vi "Main.vi"() -> ()   [LabVIEW 2020]
uses:
  <vilib>/userdefined/High Color/IMAQdx.ctl
panel:
  out "# of Matches":i32
  out "Error Out":errorcluster
  in  "Start":bool
  in  "Stop":bool
  out "# Iter":i32
  out "Image":T1(plugin-control)
  in  "Inspection Part":enum32{"P2", "P3 Top", "P3 Side"}(tab)
  out "P2 Hole":sgl
  out "P2 Left Edge Angle":sgl
  out "P2 Right Edge Angle":sgl
  out "P2 Hole Status":bool
  out "P2 Left Edge Angle Status":bool
  out "P2 Right Edge Angle Status":bool
  out "P2 Status":bool
  # "Smart Vision System Testbench"
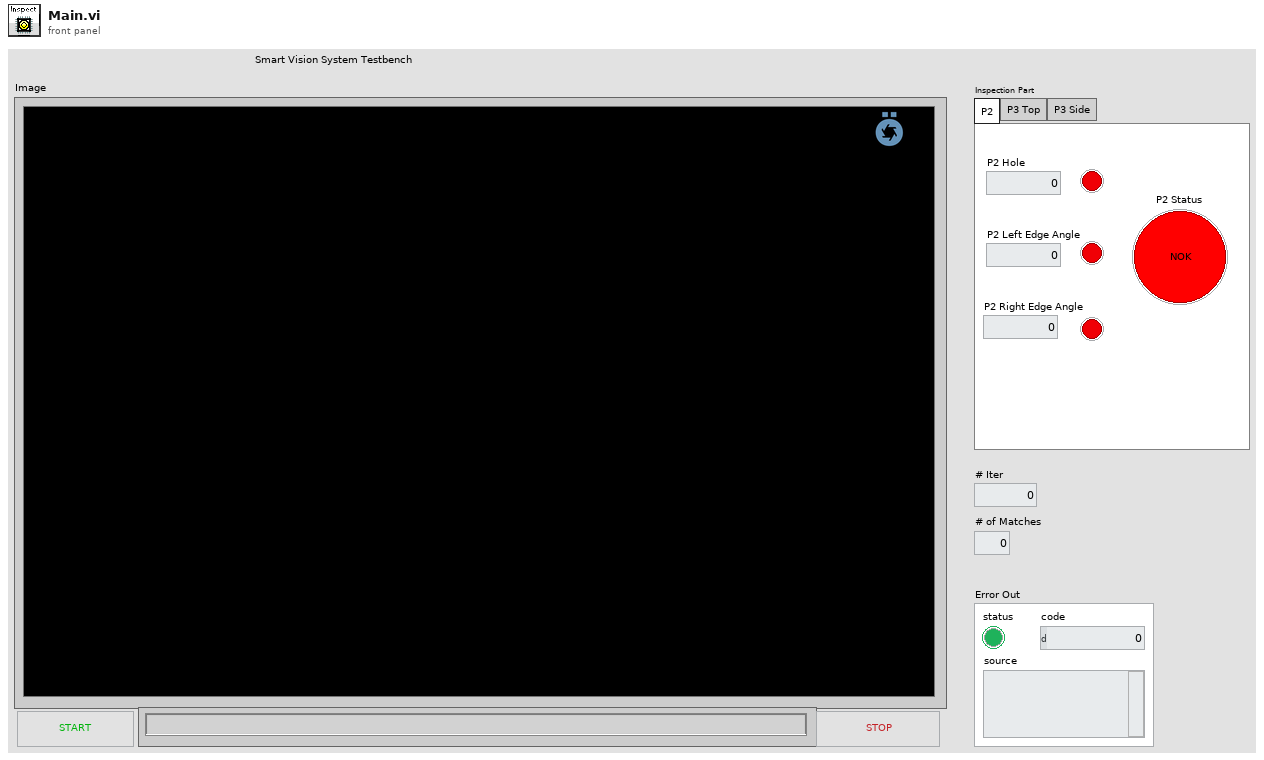
[diagram p1: front panel]
types:
  T1 = typedef "IMAQ Image.ctl" = refnum<image>
  T2 = typedef "IMAQdx.ctl" = refnum<k21>
  T3 = typedef "Image Type" = u32
  T4 = cluster{"Desired Font (Application)":enum16{"User-specified Font", "Application Font", "System Font", "Dialog Font"}, "[User-specified Font]":cluster{"Font Name":string, "Size":i16, "Strikeout?":bool, "Italic?":bool, "Underline?":bool, "Outline?":bool, "Shadow?":bool, "Bold?":bool, "Rotation Angle":dbl}, "Horizontal Alignment":i16, "Vertical Alignment":i16}
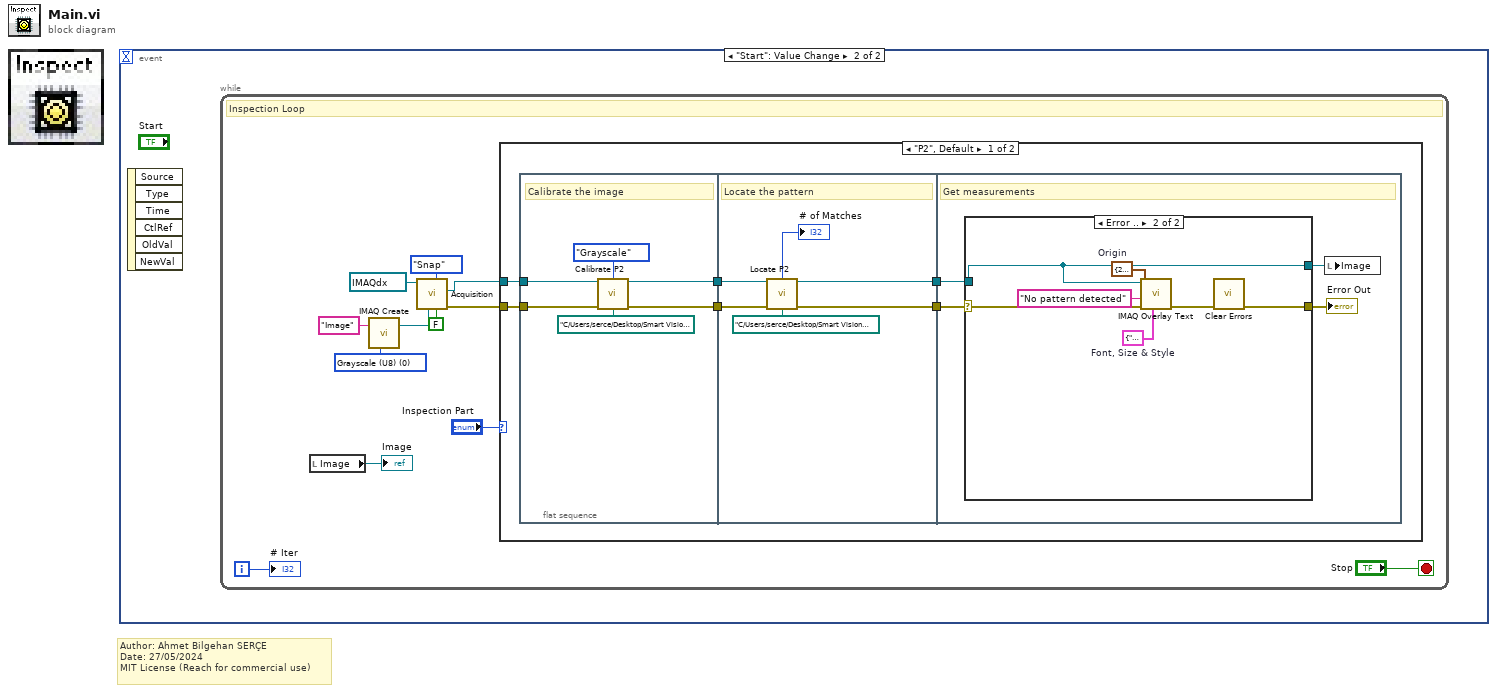
[diagram p0: block diagram]
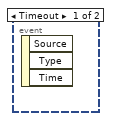
[diagram p2: hidden frame]
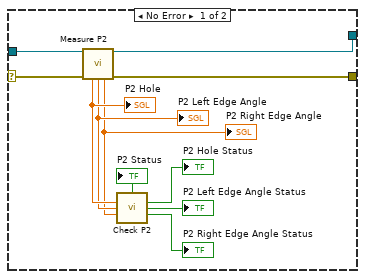
[diagram p3: hidden frame]
diagram:
  # "Author: Ahmet Bilgehan SERÇE\nDate: 27/05/2024\nMIT License (Reach for commercial use)"
  n1 = event shown="[1] \"Start\": Value Change" {
    selector: _ -> [_ _]
    dyn-events: _ -> [_ _]
    timeout: _ -> [_ _]
    event Timeout {
      n2 = event-data() -> ()  [unwired: 1 in, 3 out]
    }
    event "Start": Value Change {
      n3 = event-data() -> ()  [unwired: 1 in, 6 out]
      n4 = while {
        i -> [w12]
        stop <- "Stop" stop-if-true
        w9 = T3 0 items=["Grayscale (U8)", "Grayscale (I16)", "Grayscale (SGL)", "Complex (CSG)", "RGB (U32)", "HSL (U32)", "RGB (U64)", "Grayscale (U16)"] ("Image Type")
        # "Inspection Loop"
        n5 = local read "Image"() -> (→"Image":T1)
        n6 = call "IMAQ Create"("Image Name"="Image", "Image Type"=w9) -> ("New Image"=w8:T1)  [unwired: 3 in, 1 out]
        n7 = call "Acquisition.vi"("Set Params?"=FALSE, "Mode"=enum16{"Grab", "Snap"}."Snap", "Image Reference"=w8, "Session In"=T2 "cam5") -> ("Error Out"=w5:errorcluster, "Image Out"=w6:T1)  [unwired: 5 in, 1 out]
        n8 = case shown="\"P2\", Default" "Inspection Part" {
          tunnel: w6 -> [w14 _]
          tunnel: w5 -> [w13 _]
          frame "P2", Default {
            n9 = flat-sequence {
              tunnel: w14 -> [w24]
              tunnel: w13 -> [w23]
              tunnel: [w21] -> w18
              tunnel: [w20] -> w17
              tunnel: w18 -> [w30]
              tunnel: w17 -> [w29]
              tunnel: [w26] -> w16
              tunnel: [w25] -> w15
              tunnel: w16 -> [w33]
              tunnel: w15 -> [w34]
              frame #0 {
                # "Calibrate the image"
                n10 = call "Calibrate P2.vi"("Image In"=w24, "Image Type"=enum16{"RGB", "Grayscale"}."Grayscale", "Error In"=w23, "File Path (Image Calibration P2)"=path "C:/Users/serce/Desktop/Smart Vision System Testbench/Grid Calibration.png") -> ("Corrected Image"=w21:T1, "Error Out"=w20:errorcluster)  [unwired: 10 in]
              }
              frame #1 {
                # "Locate the pattern"
                n11 = call "Locate P2.vi"("Image In"=w30, "Error In"=w29, "Template File Path (Locate P2 Hole)"=path "C:/Users/serce/Desktop/Smart Vision System Testbench/P2/P2 Hole Template.png") -> ("Number of Matches (Locate P2 Hole)"=→"# of Matches":i32, "Image Dup Out"=w26:T1, "Error Out"=w25:errorcluster)  [unwired: 10 in]
              }
              frame #2 {
                # "Get measurements"
                n12 = case shown="Error .." w34 {
                  selector: w34 -> [w37 w52]
                  tunnel: w33 -> [w38 w51]
                  tunnel: [w36 w51] -> w32
                  tunnel: [w35 w46] -> w31
                  frame No Error {
                    n13 = call "Measure P2.vi"("Image Dup In"=w38, "Error In"=w37) -> ("Image Out"=w36:T1, "Calibrated Results (P2 Hole)"=w45:sgl, "Calibrated Results (P2 Left Edge Angles)"=w40:sgl, "Calibrated Results (P2 Right Edge Angle)"=w39:sgl, "Error Out"=w35:errorcluster)  [unwired: 9 in]
                    "P2 Hole" <- w45
                    "P2 Left Edge Angle" <- w40
                    "P2 Right Edge Angle" <- w39
                    n14 = call "Check P2.vi"("Calibrated Results (P2 Hole)"=w45, "Calibrated Results (P2 Right Edge Angle)"=w40, "Calibrated Results (P2 Left Edge Angles)"=w39) -> ("P2 Status"=→"P2 Status":bool, "P2 Hole Status"=→"P2 Hole Status":bool, "P2 Left Edge Angle Status"=→"P2 Left Edge Angle Status":bool, "P2 Right Edge Angle Status"=→"P2 Right Edge Angle Status":bool)  [unwired: 9 in]
                  }
                  frame Error {
                    w48 = T4 {"Desired Font (Application)"=enum."Application Font", "[User-specified Font]"={"Font Name"="", "Size"=20, "Strikeout?"=FALSE, "Italic?"=FALSE, "Underline?"=FALSE, "Outline?"=FALSE, "Shadow?"=FALSE, "Bold?"=FALSE, "Rotation Angle"=0.0}, "Horizontal Alignment"=0, "Vertical Alignment"=0}  # Font, Size & Style
                    w49 = cluster{"X":i32, "Y":i32} {"X"=250, "Y"=250}  # Origin
                    n15 = call "IMAQ Overlay Text"("Font, Size & Style"=w48, "error in (no error)"=w52, "String"="No pattern detected", "Origin"=w49, "Image"=w51) -> ("error out"=w47:errorcluster)  [unwired: 5 in, 1 out]
                    n16 = call <vilib>:"Clear Errors.vi"("error in (no error)"=w47) -> ("error out"=w46:errorcluster)  [unwired: 5 in, 1 out]
                  }
                }
                "Error Out" <- w31
                n17 = local write "Image"(w32) -> ()
              }
            }
          }
          frame "P3 Top" {
          }
        }
        "# Iter" <- w12
      }
    }
  }
